vi "Get Kronostamp.vy.vi"() -> (0 "kronostamp":dbl)   [LabVIEW 2020]
panel:
  out "Second":string
  out "Minute":string
  out "Hour":string
  out "time string":string
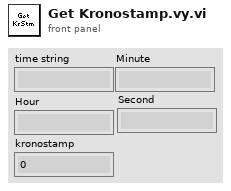
[diagram p1: front panel]
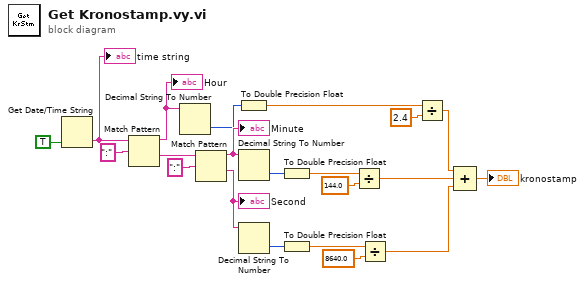
[diagram p0: block diagram]
diagram:
  n1 = Get Date/Time String(want seconds? (F)=TRUE) -> (time string=w20:string)  [unwired: 2 in, 1 out]
  "time string" <- w20
  n2 = Match Pattern(string=w20, regular expression=":") -> (before substring=w16:string, after substring=w17:string)  [unwired: 1 in, 2 out]
  "Hour" <- w16
  n3 = Decimal String To Number(string=w16) -> (number=w13:i32)  [unwired: 2 in, 1 out]
  n4 = Match Pattern(string=w17, regular expression=":") -> (before substring=w15:string, after substring=w14:string)  [unwired: 1 in, 2 out]
  "Minute" <- w15
  "Second" <- w14
  n5 = To Double Precision Float(number=w13) -> (double precision float=w8:dbl)
  n6 = Decimal String To Number(string=w15) -> (number=w12:i32)  [unwired: 2 in, 1 out]
  n7 = Decimal String To Number(string=w14) -> (number=w11:i32)  [unwired: 2 in, 1 out]
  n8 = To Double Precision Float(number=w12) -> (double precision float=w9:dbl)
  n9 = To Double Precision Float(number=w11) -> (double precision float=w10:dbl)
  n10 = Divide(x=w9, y=144.0) -> (x/y=w2:dbl)
  n11 = Divide(x=w10, y=8640.0) -> (x/y=w3:dbl)
  n12 = Divide(x=w8, y=2.4) -> (x/y=w6:dbl)
  n13 = Compound Arithmetic op=ADD(w6, w2, w3) -> (→"kronostamp":dbl)
